vi "Cluster Controls to Strings.vi"(0 "Controls[]":refnum<vi>[](array[refnum]), 11 "Error In":errorcluster) -> (4 "Control Labels":string[](array[string]), 6 "Control Values":string[](array[string]), 15 "Error Out":errorcluster)   [LabVIEW 2013]
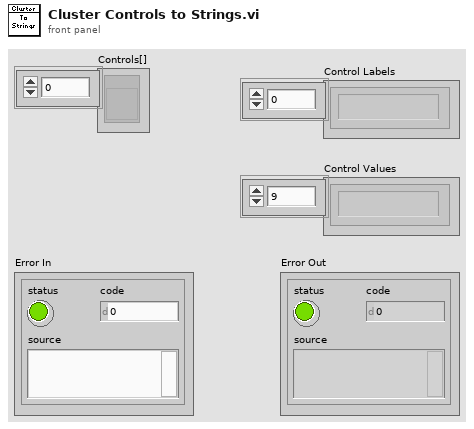
[diagram p1: front panel]
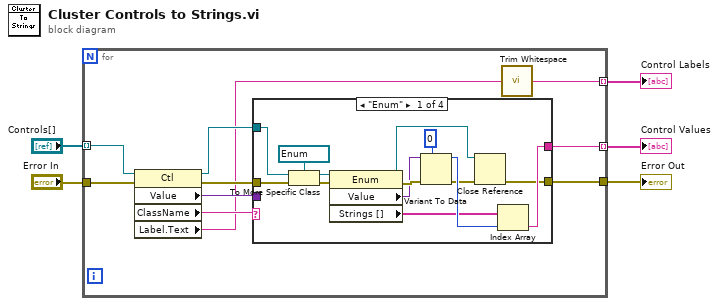
[diagram p0: block diagram]
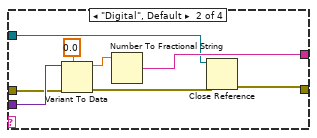
[diagram p2: hidden frame]
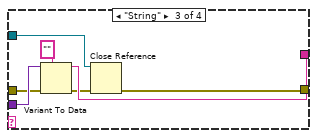
[diagram p3: hidden frame]
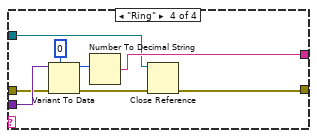
[diagram p4: hidden frame]
diagram:
  n1 = for {
    tunnel: "Controls[]" -> [w15] mode=indexing
    tunnel: [w6] -> w5 mode=indexing
    tunnel: "Error In" -> [w14]
    tunnel: [w10] -> w3 mode=indexing
    tunnel: [w8] -> w1
    n2 = property class="Ctl"(reference=w15, error in=w14) -> (reference out=w11:refnum<vi>, error out=w9:errorcluster, "Value"=w13:variant, "ClassName"=w12:string, "Label.Text"=w7:string)
    n3 = case shown="\"Enum\"" w12 {
      tunnel: [w21 w35 w43 w50] -> w10
      tunnel: [w17 w32 w38 w47] -> w8
      tunnel: w13 -> [_ w34 w42 w49]
      tunnel: w11 -> [w20 w30 w40 w45]
      tunnel: w9 -> [w19 w33 w39 w48]
      frame "Enum" {
        n4 = To More Specific Class(target class=refnum<vi> refnum ("TESTITEM"), reference=w20, error in=w19) -> (specific class reference=w23:refnum<vi>, error out=w24:errorcluster)
        n5 = property class="Enum"(reference=w23, error in=w24) -> (reference out=w16:refnum<vi>, error out=w29:errorcluster, "Value"=w26:variant, "Strings []"=w25:string[])
        n6 = Variant To Data(error in=w29, type=0 ("Index"), Variant=w26) -> (data=w28:i32, error out=w18:errorcluster)
        n7 = Close Reference(reference=w16, error in (no error)=w18) -> (error out=w17:errorcluster)
        n8 = Index Array(array=w25, index=w28) -> (element=w21:string)
      }
      frame "Digital", Default {
        n9 = Variant To Data(error in=w33, type=0.0, Variant=w34) -> (data=w36:dbl, error out=w31:errorcluster)
        n10 = Number To Fractional String(number=w36) -> (F-format string=w35:string)  [unwired: 3 in]
        n11 = Close Reference(reference=w30, error in (no error)=w31) -> (error out=w32:errorcluster)
      }
      frame "String" {
        n12 = Variant To Data(error in=w39, type="", Variant=w42) -> (data=w43:string, error out=w41:errorcluster)
        n13 = Close Reference(reference=w40, error in (no error)=w41) -> (error out=w38:errorcluster)
      }
      frame "Ring" {
        n14 = Variant To Data(error in=w48, type=0, Variant=w49) -> (data=w51:i32, error out=w46:errorcluster)
        n15 = Number To Decimal String(number=w51) -> (decimal integer string=w50:string)  [unwired: 1 in]
        n16 = Close Reference(reference=w45, error in (no error)=w46) -> (error out=w47:errorcluster)
      }
    }
    n17 = call <vilib>:"Trim Whitespace.vi"("string"=w7) -> ("trimmed string"=w6:string)  [unwired: 1 in]
  }
  "Control Values" <- w3
  "Control Labels" <- w5
  "Error Out" <- w1
